vi "Remove Aliases.vi"(8 "Error in":errorcluster, 11 "Runtime Configuration Ref in":refnum<k24>) -> (0 "Error out":errorcluster, 3 "Runtime Configuration Ref out":refnum<k24>)   [LabVIEW 2026, in "NIVS Runtime Configuration File Scripting API.lvlib"]
uses:
  NIVS Runtime Configuration File Scripting API.lvlib
  NationalInstruments.VeriStand.SystemDefinitionAPI
  <vilib>/NI/NI VeriStand Runtime Configuration File API/Runtime Configuration File API.lvlib
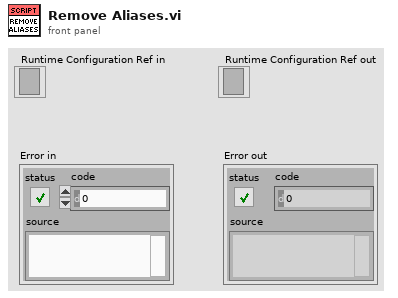
[diagram p1: front panel]
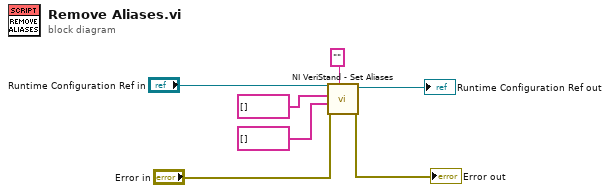
[diagram p0: block diagram]
diagram:
  n1 = call <vilib>:"NI VeriStand - Set Aliases.vi"("Runtime Alias Folder Name"="", "Error in"="Error in", "Alias Names"=string[] [], "Referenced Channels"=string[] [], "Runtime Configuration Ref in"="Runtime Configuration Ref in") -> ("Error out"=→"Error out":errorcluster, "Runtime Configuration Ref out"=→"Runtime Configuration Ref out":refnum<k24>)  [unwired: 4 in, 1 out]
